vi "Call_SubPanal.vi"(8 "错误输入（无错误）":errorcluster, 10 "VI引用句柄":refnum<vi>, 11 "SubPnl引用句柄":refnum<vi>) -> (0 "错误输出":errorcluster)   [LabVIEW 2018]
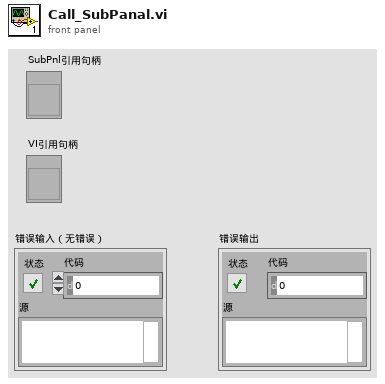
[diagram p1: front panel]
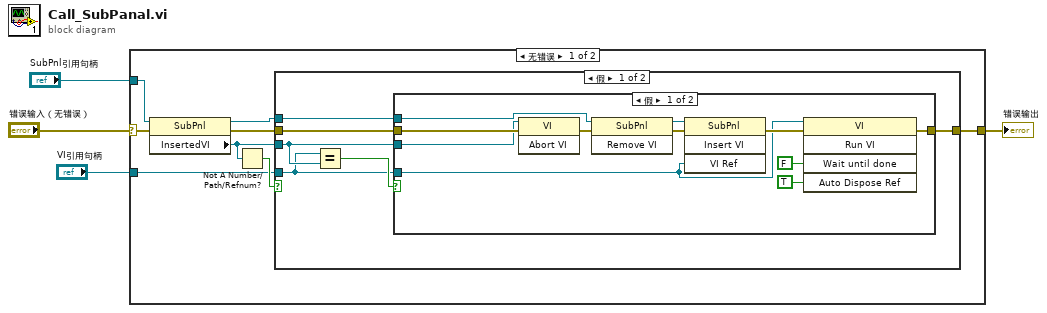
[diagram p0: block diagram]
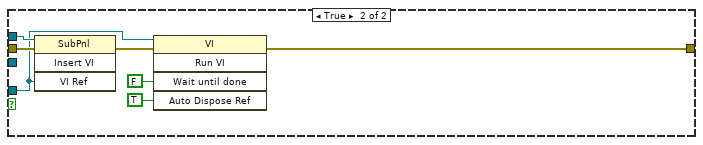
[diagram p3: hidden frame]
diagram:
  n1 = case shown="无错误" "错误输入（无错误）" {
    selector: "错误输入（无错误）" -> [w7 w38]
    tunnel: "SubPnl引用句柄" -> [w8 _]
    tunnel: "VI引用句柄" -> [w6 _]
    tunnel: [w5 w38] -> w1
    frame No Error {
      n2 = property class="SubPnl"(reference=w8, error in=w7) -> (reference out=w10:refnum<vi>, error out=w9:errorcluster, "InsertedVI"=w11:refnum<vi>)
      n3 = Not A Number/Path/Refnum?(number/path/refnum=w11) -> (NaN/Path/Refnum?=w12:bool)
      n4 = case shown="假" w12 {
        tunnel: w11 -> [w16 _]
        tunnel: w10 -> [w18 w36]
        tunnel: w9 -> [w17 w37]
        tunnel: w6 -> [w14 w34]
        tunnel: [w13 w31] -> w5
        frame False {
          n5 = Equal?(x=w14, y=w16) -> (x = y?=w15:bool)
          n6 = case shown="假" w15 {
            tunnel: w18 -> [w29 _]
            tunnel: w17 -> [w27 w30]
            tunnel: w16 -> [w26 _]
            tunnel: w14 -> [w22 _]
            tunnel: [w19 w30] -> w13
            frame False {
              n7 = invoke class="VI" method="Abort VI"(reference=w26, error in=w27) -> (error out=w28:errorcluster)  [unwired: 1 in, 2 out]
              n8 = invoke class="SubPnl" method="Remove VI"(reference=w29, error in=w28) -> (reference out=w24:refnum<vi>, error out=w25:errorcluster)  [unwired: 1 in, 1 out]
              n9 = invoke class="SubPnl" method="Insert VI"(reference=w24, error in=w25, "VI Ref"=w22) -> (error out=w23:errorcluster)  [unwired: 1 in, 3 out]
              n10 = invoke class="VI" method="Run VI"(reference=w22, error in=w23, "Wait until done"=FALSE ("结束前等待"), "Auto Dispose Ref"=TRUE ("自动销毁引用")) -> (error out=w19:errorcluster)  [unwired: 1 in, 4 out]
            }
            frame True {
            }
          }
        }
        frame True {
          n11 = invoke class="SubPnl" method="Insert VI"(reference=w36, error in=w37, "VI Ref"=w34) -> (error out=w35:errorcluster)  [unwired: 1 in, 3 out]
          n12 = invoke class="VI" method="Run VI"(reference=w34, error in=w35, "Wait until done"=FALSE ("结束前等待"), "Auto Dispose Ref"=TRUE ("自动销毁引用")) -> (error out=w31:errorcluster)  [unwired: 1 in, 4 out]
        }
      }
    }
    frame Error {
    }
  }
  "错误输出" <- w1
